vi "Get Tool.vi"(8 "error in (no error)":errorcluster, 10 "Name":string, 11 "id in":i32) -> (0 "error out":errorcluster, 1 "found?":bool, 2 "Tool Data":T1, 3 "id out":i32)   [LabVIEW 2025, in "MCP Server.lvlib"]
uses:
  MCP Server.lvlib
  Tool Data.ctl
  Input Parameter.ctl
  Output Parameter.ctl
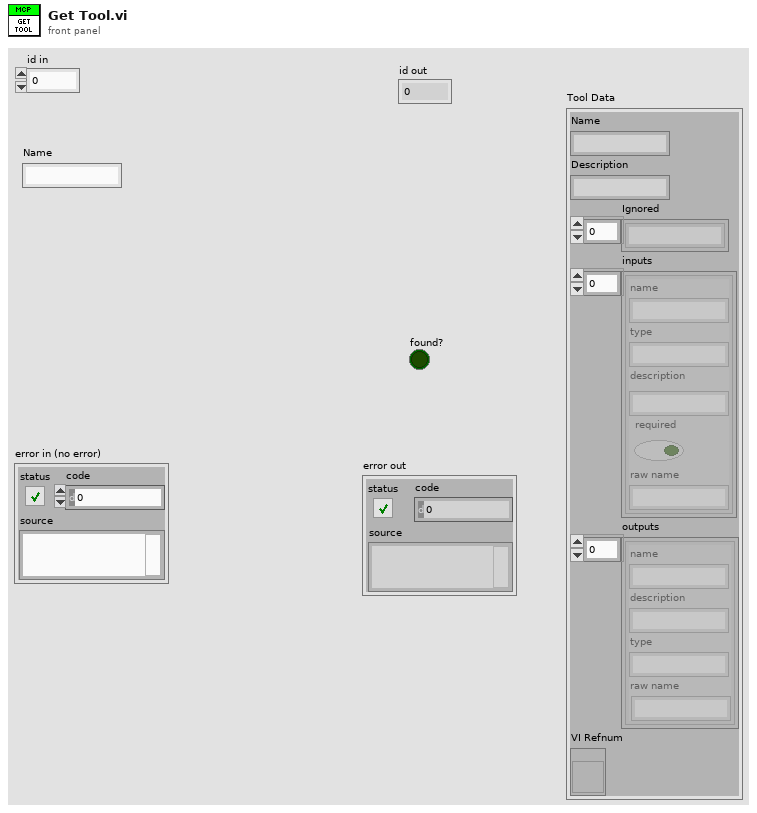
[diagram p1: front panel]
types:
  T1 = typedef "MCP Server.lvlib/Tool Data.ctl" = cluster{"Name":string, "Description":string, "Ignored":string[], "inputs":T2[], "outputs":T3[], "VI Refnum":refnum<vi>}
  T2 = typedef "MCP Server.lvlib/Input Parameter.ctl" = cluster{"name":string, "type":string, "description":string, "required":bool, "raw name":string}
  T3 = typedef "MCP Server.lvlib/Output Parameter.ctl" = cluster{"name":string, "description":string, "type":string, "raw name":string}
  T4 = typedef "MCP Server.lvlib/Server Data.ctl" = cluster{"Name":string, "Description":string, "Tools":T1[], "Parameters":string[][], "Logging Info":T5, "User Events":T6, "Prompts":T7[], "resources":T9[], "HTTP Server":refnum<class "Server.lvclass">}
  T5 = typedef "MCP Server.lvlib/Logging.ctl" = cluster{"Log":string[], "Max Length":i32}
  T6 = typedef "MCP Server.lvlib/User Events.ctl" = cluster{"onError":refnum<user-event>, "onRpc":refnum<user-event>}
  T7 = typedef "MCP Server.lvlib/Prompt Data.ctl" = cluster{"name":string, "description":string, "arguments":T8[], "return terminal name":string, "results description":string, "VI Refnum":refnum<vi>}
  T8 = typedef "MCP Server.lvlib/Prompt Argument.ctl" = cluster{"name":string, "description":string, "required":bool, "raw_name":string}
  T9 = typedef "MCP Server.lvlib/resource data.ctl" = cluster{"uri":string, "name":string, "description":string, "mimeType":string, "file path":path}
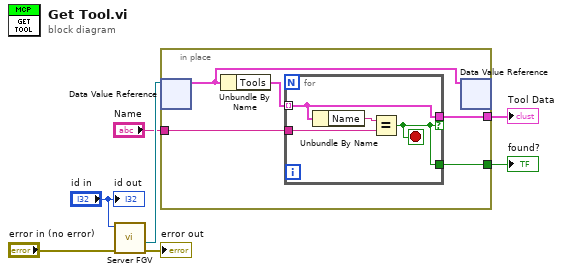
[diagram p0: block diagram]
diagram:
  n1 = call "Server FGV.vi"("error in"="error in (no error)", "id"="id in") -> ("error out"=→"error out":errorcluster, "server reference"=w4:refnum<data-value>)  [unwired: 5 in, 3 out]
  n2 = in-place {
    in-place-border: "Name" -> [w11]
    in-place-border: [w9] -> w2
    in-place-border: [w8] -> w1
    n3 = in-place-dvr #1(w4) -> (w10:T4)  [unwired: 1 out]
    n4 = Unbundle By Name(w10) -> ("Tools"=w12:T1[])
    n5 = for {
      tunnel: w12 -> [w14] mode=indexing
      tunnel: w11 -> [w15]
      tunnel: [w14] -> w9 if=w13
      tunnel: [w13] -> w8
      stop <- w13 stop-if-true
      n6 = Unbundle By Name(w14) -> ("Name"=w16:string)
      n7 = Equal?(x=w16, y=w15) -> (x = y?=w13:bool)
    }
    n8 = in-place-dvr #1(w10) -> ()  [unwired: 2 out]
  }
  "Tool Data" <- w2
  "found?" <- w1
  "id out" <- "id in"
